vi "LanguagesSettings.vi"() -> ()   [LabVIEW 2013]
panel:
  out "LanguageSettings":T1
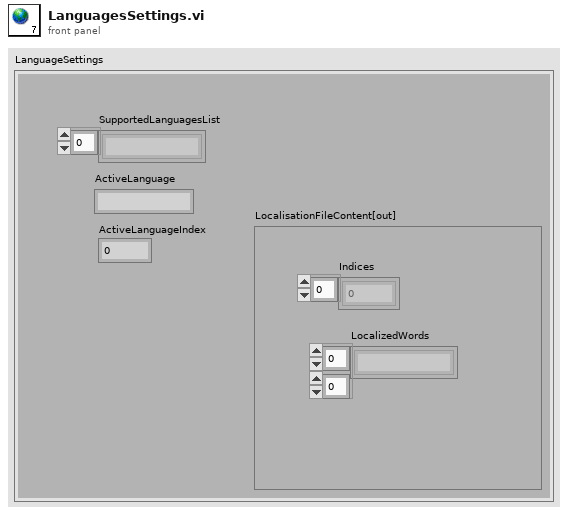
[diagram p1: front panel]
types:
  T1 = cluster{"SupportedLanguagesList":string[], "ActiveLanguage":string, "ActiveLanguageIndex":u16, "LocalisationFileContent[out]":cluster{"Indices":u32[], "LocalizedWords":string[][]}}
diagram:
